vi "testRunCalledForEachTestCase.vi"() -> (0 "error out":errorcluster)   [LabVIEW 2019, in "TestSuiteTest.lvlib" / "Run.lvlib"]
uses:
  Run.lvlib
  TestSuite/TestSuite.lvclass
  TestCase/TestCase/TestCase.lvclass
  TestSuiteTestSupport/TestResultMock/TestResultMock.lvclass
  C:/Users/de200256/Code/LVUnit/TestResult/TestResult.lvclass
  Assertion/Assertion.lvlib
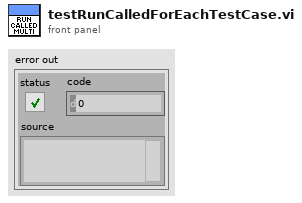
[diagram p1: front panel]
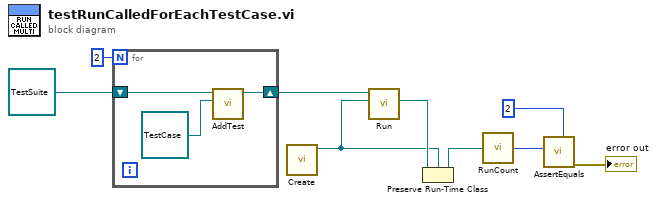
[diagram p0: block diagram]
diagram:
  n1 = for {
    N: 2 -> [_]
    shift-right: [w11] -> w4
    shift-left: refnum<class "TestSuite.lvclass"> refnum ("TestSuite.lvclass") -> [w12]
    n2 = call-dynamic "AddTest.vi"("TestCase"=refnum<class "TestCase.lvclass"> refnum, "TestSuite in"=w12) -> ("TestSuite out"=w11:refnum<class "TestSuite.lvclass">)  [unwired: 8 in, 1 out]
  }
  n3 = call "Create.vi"() -> ("TestResultMock"=w8:refnum<class "TestResultMock.lvclass">)  [unwired: 10 in, 1 out]
  n4 = call-dynamic "Run.vi"("TestResult"=w8, "TestSuite in"=w4) -> ("TestResult out"=w9:refnum<class "TestResult.lvclass">)  [unwired: 7 in, 2 out]
  n5 = Preserve Run-Time Class(object in=w9, 2:w8) -> (object out=w7:refnum<class "TestResultMock.lvclass">)  [unwired: 1 in, 1 out]
  n6 = call "RunCount.vi"("TestResultMock In"=w7) -> ("Run Count"=w6:i32)
  n7 = call "AssertEquals.vi"("Expected"=2 ("Run Count"), "Actual"=w6) -> ("error out"=→"error out":errorcluster)  [unwired: 9 in]
